vi "Binary Division.vi"(10 "Divisor (Binary)":i32 format="%b", 11 "Dividend (Binary)":i32 format="%b") -> (2 "Remainder  (Binary)":i32 format="%b", 3 "Quotient  (Binary)":i32 format="%b")   [LabVIEW 2020]
doc: "This VI will divide two Binary Numbers and will be ouputing respective Quotient and Remainder."
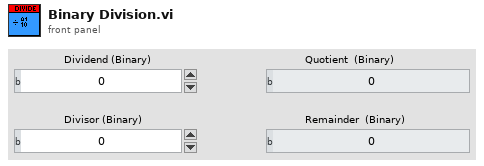
[diagram p1: front panel]
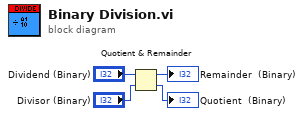
[diagram p0: block diagram]
diagram:
  n1 = Quotient & Remainder(x="Dividend (Binary)", y="Divisor (Binary)") -> (x-y*floor(x/y)=→"Remainder  (Binary)":i32, floor(x/y)=→"Quotient  (Binary)":i32)
